vi "State_Machine.vi"() -> ()   [LabVIEW 2018]
uses:
  <vilib>/Utility/file.llb/Write Delimited Spreadsheet (string).vi
  <vilib>/Utility/file.llb/Read Delimited Spreadsheet (string).vi
panel:
  out "unsuccessful attemp # 2":i32=3
  in  "OK Button":bool
  in  "Admin Pass for lock out":string
  out "Yellow 2":bool
  out "unsuccessful attemp #":i32=3
  in  "stop":bool
  out "x = y?":bool
  out "Error Message":string
  out "red":bool
  out "File Directory":path
  in  "Search":bool
  in  "PIN":string
  in  "OU_ID":string
  in  "NAME":string
  # "File Directory = Where my files are \nlocated inside the pc."
  # "SHIT ROOM STATEMACHINE"
  # "Yellow LED for searched successful ==>\nRed LED for search unsuccessful      ==>"
  # "untill an administrative password is supplied.\n\nFeature creep:\n4) admin password -- changes alot\n3) successful fcked up"
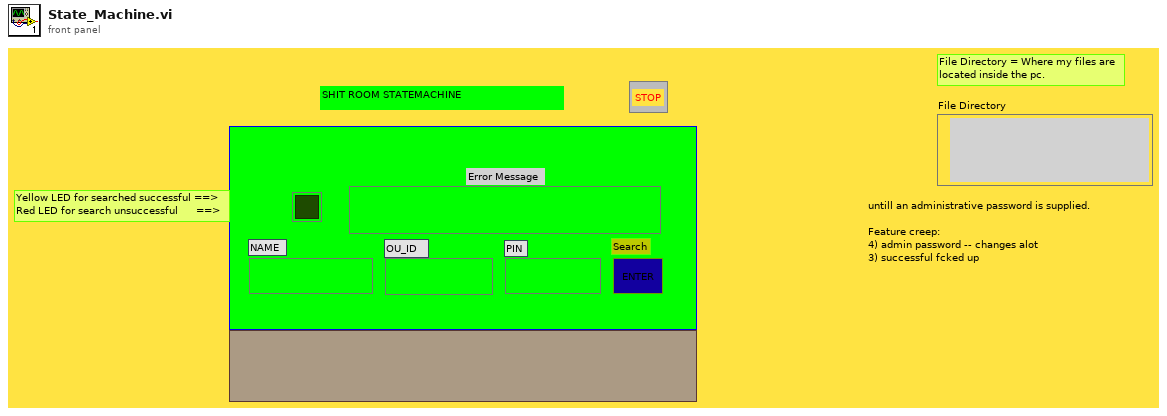
[diagram p1: front panel]
types:
  T1 = enum8{"Enabled", "Disabled", "Disabled and Grayed Out"}
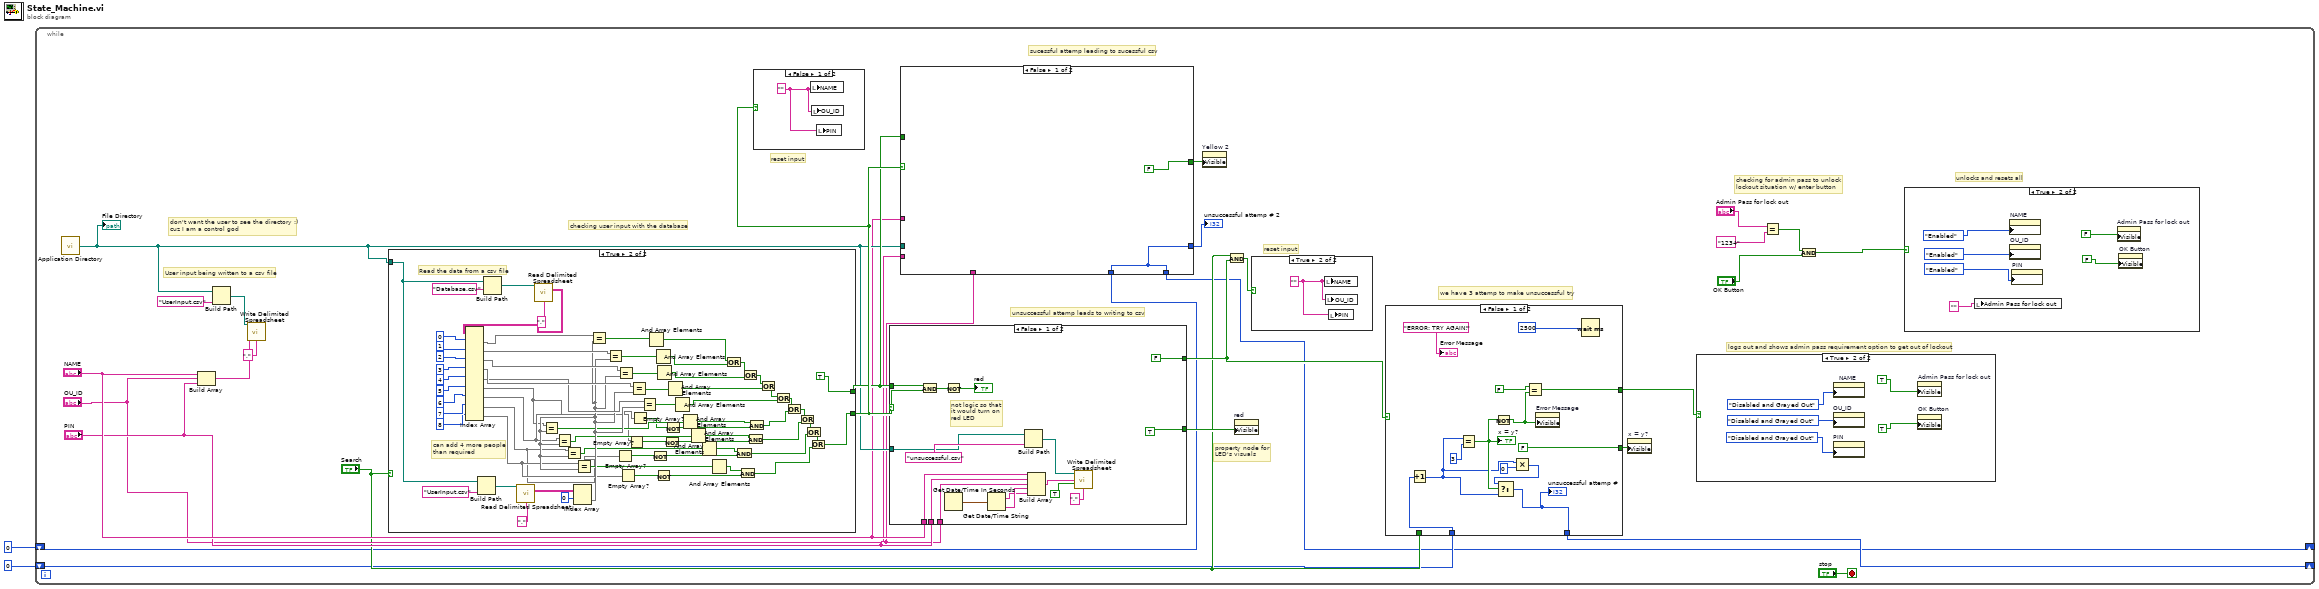
[diagram p0: block diagram]
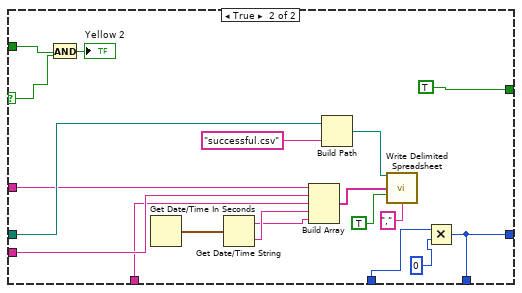
[diagram p2: hidden frame]
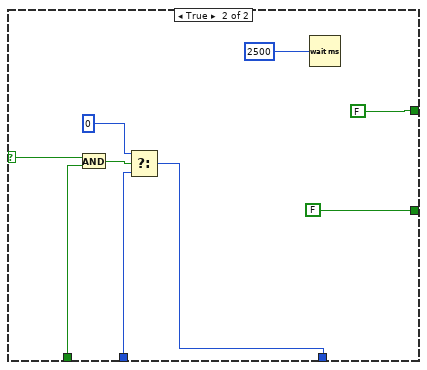
[diagram p7: hidden frame]
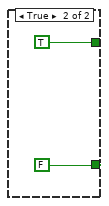
[diagram p8: hidden frame]
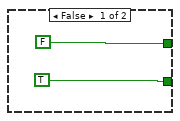
[diagram p9: hidden frame]
diagram:
  n1 = while {
    shift-right: [w4] -> _
    shift-left: 0 -> [w5]
    shift-right: [w14] -> _
    shift-left: 0 -> [w6]
    stop <- "stop" stop-if-true
    # "unlocks and resets all"
    # "checking for admin pass to unlock\nlockout situation w/ enter button"
    # "logs out and shows admin pass requirement option to get out of lockout"
    # "we have 3 attemp to make unsuccessful try"
    # "reset input"
    # "reset input"
    # "checking user input with the database"
    # "sucessful attemp leading to sucessful csv"
    # "unsuccessful attemp leads to writing to csv"
    # "don't want the user to see the directory :)\ncuz I am a control god"
    # "property node for\nLED's visuals"
    # "User input being written to a csv file"
    n2 = call <vilib>:"Application Directory.vi"() -> ("Application Directory"=w20:path)
    "File Directory" <- w20
    n3 = Build Array("NAME", "OU_ID", "PIN") -> (w29:string[])
    n4 = Build Path(base path=w20, name or relative path="UserInput.csv") -> (appended path=w26:path)
    n5 = call-poly <vilib>:"Write Delimited Spreadsheet.vi"("file path (dialog if empty)"=w26, "1D data"=w29, "delimiter (\\t)"=",") -> ()  [unwired: 11 in, 2 out]
    n6 = case shown="True" "Search" {
      tunnel: w20 -> [_ w167]
      tunnel: [TRUE w130] -> w22
      tunnel: [FALSE TRUE] -> w21
      frame False {
      }
      frame True {
        # "can add 4 more people \nthan required"
        # "Read the data from a csv file"
        n7 = Build Path(base path=w167, name or relative path="UserInput.csv") -> (appended path=w171:path)
        n8 = Build Path(base path=w167, name or relative path="Database.csv") -> (appended path=w175:path)
        n9 = call-poly <vilib>:"Read Delimited Spreadsheet.vi"("file path (dialog if empty)"=w171, "delimiter (\\t)"="," ("delimiter (\\t)")) -> ("all rows"=w169:string[][])  [unwired: 8 in, 5 out]
        n10 = call-poly <vilib>:"Read Delimited Spreadsheet.vi"("file path (dialog if empty)"=w175, "delimiter (\\t)"="," ("delimiter (\\t)")) -> ("all rows"=w165:string[][])  [unwired: 8 in, 5 out]
        n11 = Index Array(array=w165, index (row) #1=0 ("index"), index (row) #2=1 ("index"), index (row) #3=2 ("index"), index (row) #4=3 ("index"), index (row) #5=4 ("index"), index (row) #6=5 ("index"), index (row) #7=6 ("index"), index (row) #8=7 ("index"), index (row) #9=8 ("index")) -> (element #1=w160:string[], element #2=w159:string[], element #3=w158:string[], element #4=w157:string[], element #5=w139:string[], element #6=w109:string[], element #7=w116:string[], element #8=w121:string[], element #9=w128:string[])  [unwired: 9 in]
        n12 = Index Array(array=w169, index (row)=0 ("index")) -> (element=w138:string[])  [unwired: 1 in]
        n13 = Equal?(x=w109, y=w138) -> (x = y?=w137:bool[])
        n14 = Equal?(x=w116, y=w138) -> (x = y?=w136:bool[])
        n15 = Equal?(x=w121, y=w138) -> (x = y?=w135:bool[])
        n16 = Equal?(x=w128, y=w138) -> (x = y?=w129:bool[])
        n17 = Equal?(x=w160, y=w138) -> (x = y?=w154:bool[])
        n18 = Equal?(x=w159, y=w138) -> (x = y?=w152:bool[])
        n19 = Empty Array?(array=w121) -> (empty?=w123:bool)
        n20 = Equal?(x=w158, y=w138) -> (x = y?=w150:bool[])
        n21 = Empty Array?(array=w128) -> (empty?=w125:bool)
        n22 = Empty Array?(array=w116) -> (empty?=w118:bool)
        n23 = Equal?(x=w157, y=w138) -> (x = y?=w147:bool[])
        n24 = Empty Array?(array=w109) -> (empty?=w113:bool)
        n25 = Equal?(x=w139, y=w138) -> (x = y?=w145:bool[])
        n26 = And Array Elements(Boolean array=w154) -> (logical AND=w153:bool)
        n27 = Not(x=w123) -> (.not. x?=w122:bool)
        n28 = And Array Elements(Boolean array=w152) -> (logical AND=w151:bool)
        n29 = Not(x=w125) -> (.not. x?=w124:bool)
        n30 = And Array Elements(Boolean array=w150) -> (logical AND=w149:bool)
        n31 = Not(x=w118) -> (.not. x?=w117:bool)
        n32 = Not(x=w113) -> (.not. x?=w112:bool)
        n33 = And Array Elements(Boolean array=w147) -> (logical AND=w146:bool)
        n34 = And Array Elements(Boolean array=w145) -> (logical AND=w144:bool)
        n35 = And Array Elements(Boolean array=w137) -> (logical AND=w111:bool)
        n36 = And Array Elements(Boolean array=w136) -> (logical AND=w115:bool)
        n37 = And Array Elements(Boolean array=w135) -> (logical AND=w120:bool)
        n38 = And Array Elements(Boolean array=w129) -> (logical AND=w127:bool)
        n39 = Or(x=w153, y=w151) -> (x .or. y?=w148:bool)
        n40 = And(x=w120, y=w122) -> (x .and. y?=w119:bool)
        n41 = And(x=w127, y=w124) -> (x .and. y?=w126:bool)
        n42 = Or(x=w148, y=w149) -> (x .or. y?=w156:bool)
        n43 = And(x=w115, y=w117) -> (x .and. y?=w114:bool)
        n44 = And(x=w111, y=w112) -> (x .and. y?=w110:bool)
        n45 = Or(x=w156, y=w146) -> (x .or. y?=w155:bool)
        n46 = Or(x=w155, y=w144) -> (x .or. y?=w134:bool)
        n47 = Or(x=w134, y=w110) -> (x .or. y?=w133:bool)
        n48 = Or(x=w133, y=w114) -> (x .or. y?=w132:bool)
        n49 = Or(x=w132, y=w119) -> (x .or. y?=w131:bool)
        n50 = Or(x=w131, y=w126) -> (x .or. y?=w130:bool)
      }
    }
    n51 = case shown="False" w22 {
      frame False {
        w64 = ""
        n52 = local write "NAME"(w64) -> ()
        n53 = local write "OU_ID"(w64) -> ()
        n54 = local write "PIN"(w64) -> ()
      }
      frame True {
      }
    }
    n55 = case shown="False" w22 {
      selector: w22 -> [w101 _]
      tunnel: [TRUE FALSE] -> w30
      tunnel: w21 -> [w102 _]
      tunnel: "NAME" -> [w95 _]
      tunnel: "PIN" -> [w94 _]
      tunnel: "OU_ID" -> [w93 _]
      tunnel: w20 -> [w96 _]
      tunnel: [FALSE TRUE] -> w15
      frame False {
        # "not logic so that\nit would turn on\nred LED"
        n56 = And(x=w102, y=w101) -> (x .and. y?=w100:bool)
        n57 = Not(x=w100) -> (.not. x?=→"red":bool)
        n58 = Get Date/Time In Seconds() -> (seconds since 1Jan1904=w91:timestamp)
        n59 = Get Date/Time String(seconds (now)=w91) -> (date string=w89:string, time string=w90:string)  [unwired: 2 in]
        n60 = Build Path(base path=w96, name or relative path="unsuccessful.csv") -> (appended path=w98:path)
        n61 = Build Array(w95, w94, w93, w90, w89) -> (w92:string[])
        n62 = call-poly <vilib>:"Write Delimited Spreadsheet.vi"("file path (dialog if empty)"=w98, "1D data"=w92, "append to file? (new file:F)"=TRUE, "delimiter (\\t)"=",") -> ()  [unwired: 10 in, 2 out]
      }
      frame True {
      }
    }
    n63 = case shown="False" w22 {
      selector: w22 -> [_ w49]
      tunnel: w21 -> [_ w50]
      tunnel: w20 -> [_ w40]
      tunnel: "NAME" -> [_ w39]
      tunnel: "PIN" -> [_ w38]
      tunnel: "OU_ID" -> [_ w37]
      tunnel: [FALSE TRUE] -> w16
      tunnel: w5 -> [w31 w35]
      tunnel: [w31 w33] -> w4
      tunnel: [w31 w33] -> w3
      frame False {
      }
      frame True {
        n64 = And(x=w50, y=w49) -> (x .and. y?=→"Yellow 2":bool)
        n65 = Get Date/Time In Seconds() -> (seconds since 1Jan1904=w45:timestamp)
        n66 = Get Date/Time String(seconds (now)=w45) -> (date string=w43:string, time string=w44:string)  [unwired: 2 in]
        n67 = Build Array(w39, w38, w37, w44, w43) -> (w47:string[])
        n68 = Build Path(base path=w40, name or relative path="successful.csv") -> (appended path=w48:path)
        n69 = call-poly <vilib>:"Write Delimited Spreadsheet.vi"("file path (dialog if empty)"=w48, "1D data"=w47, "append to file? (new file:F)"=TRUE, "delimiter (\\t)"=",") -> ()  [unwired: 10 in, 2 out]
        n70 = Multiply(x=w35, y=0) -> (x*y=w33:i32)
      }
    }
    "unsuccessful attemp # 2" <- w3
    n71 = property on="Yellow 2" class="Bool (strict)"("Visible"=w16) -> ()  [unwired: 2 in, 2 out]
    n72 = And(x="Search", y=w15) -> (x .and. y?=w24:bool)
    n73 = property on="red" class="Bool (strict)"("Visible"=w30) -> ()  [unwired: 2 in, 2 out]
    n74 = case shown="True" w24 {
      frame False {
      }
      frame True {
        w63 = ""
        n75 = local write "NAME"(w63) -> ()
        n76 = local write "OU_ID"(w63) -> ()
        n77 = local write "PIN"(w63) -> ()
      }
    }
    n78 = case shown="False" w15 {
      selector: w15 -> [_ w83]
      tunnel: "Search" -> [_ w82]
      tunnel: [w68 w80] -> w14
      tunnel: [FALSE FALSE] -> w25
      tunnel: w6 -> [w65 w81]
      tunnel: [w66 FALSE] -> w12
      frame False {
        n79 = Increment(x=w65) -> (x+1=w69:i32)
        n80 = Equal?(x=w69, y=3) -> (x = y?=w71:bool)
        "x = y?" <- w71
        n81 = Not(x=w71) -> (.not. x?=w73:bool)
        n82 = Multiply(x=w69, y=0) -> (x*y=w70:i32)
        n83 = Select(t=w70, s=w71, f=w69) -> (s? t:f=w68:i32)
        "unsuccessful attemp #" <- w68
        n84 = Equal?(x=FALSE, y=w73) -> (x = y?=w66:bool)
        n85 = property on="Error Message" class="Str"("Visible"=w73) -> ()  [unwired: 2 in, 2 out]
        n86 = Wait (ms)(milliseconds to wait=u32 2500) -> ()  [unwired: 1 out]
        "Error Message" <- "ERROR: TRY AGAIN!"
      }
      frame True {
        n87 = And(x=w83, y=w82) -> (x .and. y?=w85:bool)
        n88 = Select(t=0, s=w85, f=w81) -> (s? t:f=w80:i32)
        n89 = Wait (ms)(milliseconds to wait=u32 2500) -> ()  [unwired: 1 out]
      }
    }
    n90 = property on="x = y?" class="Bool (strict)"("Visible"=w25) -> ()  [unwired: 2 in, 2 out]
    n91 = case shown="True" w12 {
      frame False {
      }
      frame True {
        n92 = property on="NAME" class="Str"("DisabledEnum"=T1."Disabled and Grayed Out" ("Disabled")) -> ()  [unwired: 2 in, 2 out]
        n93 = property on="OU_ID" class="Str"("DisabledEnum"=T1."Disabled and Grayed Out" ("Disabled")) -> ()  [unwired: 2 in, 2 out]
        n94 = property on="PIN" class="Str"("DisabledEnum"=T1."Disabled and Grayed Out" ("Disabled")) -> ()  [unwired: 2 in, 2 out]
        n95 = property on="Admin Pass for lock out" class="Str"("Visible"=TRUE) -> ()  [unwired: 2 in, 2 out]
        n96 = property on="OK Button" class="Bool"("Visible"=TRUE) -> ()  [unwired: 2 in, 2 out]
      }
    }
    n97 = Equal?(x="Admin Pass for lock out", y="1234") -> (x = y?=w8:bool)
    n98 = And(x=w8, y="OK Button") -> (x .and. y?=w7:bool)
    n99 = case shown="True" w7 {
      frame False {
      }
      frame True {
        n100 = local write "Admin Pass for lock out"("") -> ()
        n101 = property on="NAME" class="Str"("DisabledEnum"=T1."Enabled" ("Disabled")) -> ()  [unwired: 2 in, 2 out]
        n102 = property on="OU_ID" class="Str"("DisabledEnum"=T1."Enabled" ("Disabled")) -> ()  [unwired: 2 in, 2 out]
        n103 = property on="PIN" class="Str"("DisabledEnum"=T1."Enabled" ("Disabled")) -> ()  [unwired: 2 in, 2 out]
        n104 = property on="Admin Pass for lock out" class="Str"("Visible"=FALSE) -> ()  [unwired: 2 in, 2 out]
        n105 = property on="OK Button" class="Bool"("Visible"=FALSE) -> ()  [unwired: 2 in, 2 out]
      }
    }
  }
